vi "Call Code.vi"(8 "Error In":errorcluster, 10 "Pythonic Code":string, 11 "OPI Ref":refnum<data-value>) -> (0 "Error Out":errorcluster, 3 "OPI Ref":refnum<data-value>)   [LabVIEW 2016, in "OPI.lvclass"]
doc: "Call the python code specified by input string. This function can be used to define pure pythonic code before making function calls. Alternatively you can point to a .py file while obtaining a reference to OPI.\n\n<b>Important</b> - the methods called by OPI should not have infinite loops or other mechanisms blocking execution. This can cause a timeout on the OPI."
uses:
  OPI.lvclass
  OPI.lvclass/OPI.ctl
  <vilib>/Utility/error.llb/Error Cluster From Error Code.vi
  <vilib>/ErrorRing/Error Ring.xnode
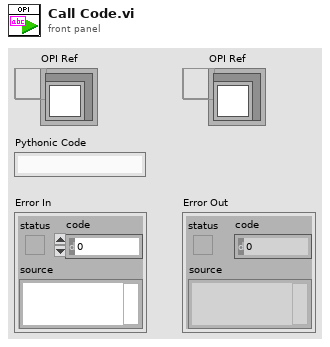
[diagram p1: front panel]
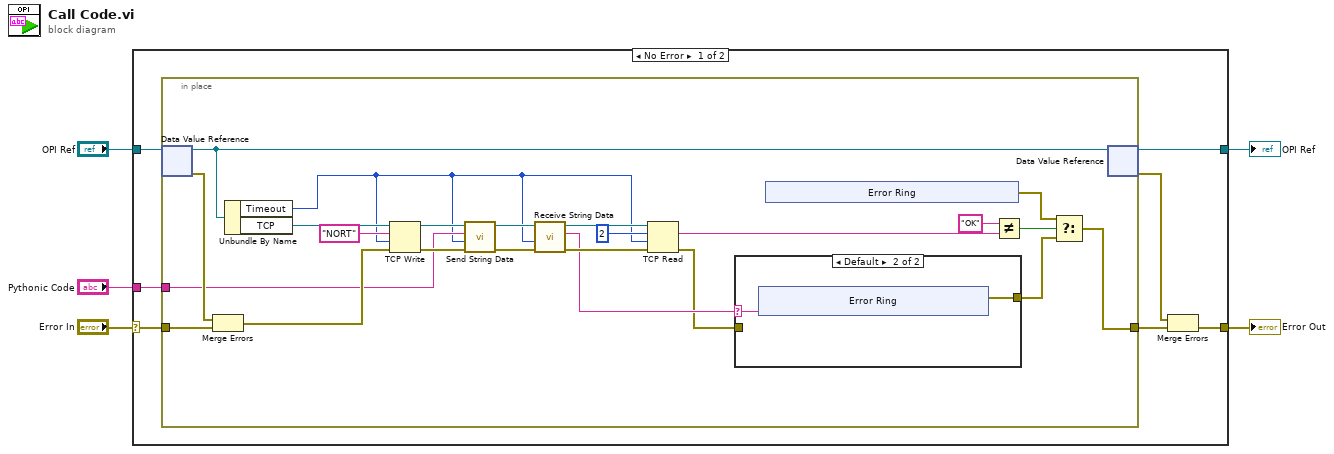
[diagram p0: block diagram]
diagram:
  n1 = case shown="No Error" "Error In" {
    selector: "Error In" -> [w12 w51]
    tunnel: [w8 w51] -> w5
    tunnel: "OPI Ref" -> [w11 w52]
    tunnel: [w10 w52] -> w2
    tunnel: "Pythonic Code" -> [w6 _]
    frame No Error {
      n2 = in-place {
        in-place-border: [w16] -> w9
        in-place-border: w12 -> [w34]
        in-place-border: w6 -> [w14]
        n3 = in-place-dvr #1(w11) -> (w15:refnum<class "OPI.lvclass">, w35:errorcluster)
        n4 = Merge Errors(w35, w34) -> (w24:errorcluster)
        n5 = Unbundle By Name(w15) -> ("Timeout"=w13:i32, "TCP"=w25:refnum<k5>)
        n6 = TCP Write(connection ID=w25, data in="NORT", error in (no error)=w24, 9:w13) -> (connection ID out=w27:refnum<k5>, error out=w28:errorcluster)  [unwired: 1 out]
        n7 = call "Send String Data.vi"("Error In"=w28, "timeout ms (25000)"=w13, "String Data"=w14, "TCP In"=w27) -> ("Error Out"=w33:errorcluster, "TCP Out"=w32:refnum<k5>)  [unwired: 6 in]
        n8 = call "Receive String Data.vi"("Error In"=w33, "timeout ms (25000)"=w13, "TCP In"=w32) -> ("Error Out"=w30:errorcluster, "String Data"=w23:string, "TCP Out"=w29:refnum<k5>)  [unwired: 6 in]
        n9 = TCP Read(connection ID=w29, bytes to read=2, error in (no error)=w30, 9:w13) -> (data out=w21:string, error out=w22:errorcluster)  [unwired: 1 in, 1 out]
        n10 = case shown="Default" w23 {
          selector: w23 -> [_ w43]
          tunnel: [w41 w42] -> w17
          tunnel: w22 -> [w41 _]
          frame "None" {
          }
          frame Default {
            n11 = xnode "Error Ring"("parameter 0"=w43) -> ("error out"=w42:errorcluster)
          }
        }
        n12 = xnode "Error Ring"() -> ("error out"=w18:errorcluster)
        n13 = Not Equal?(x="OK", y=w21) -> (x != y?=w19:bool)
        n14 = Select(t=w18, s=w19, f=w17) -> (s? t:f=w16:errorcluster)
        n15 = in-place-dvr #1(w15) -> (w10:refnum<data-value>, w7:errorcluster)
      }
      n16 = Merge Errors(w7, w9) -> (w8:errorcluster)
    }
    frame Error {
    }
  }
  "Error Out" <- w5
  "OPI Ref" <- w2
